vi "Save-buffered-GUI-values-to-file.vi"(8 "error in":errorcluster, 11 "Data ref. in":refnum<data-value>) -> (0 "error IO":errorcluster, 3 "Data ref.":refnum<data-value>)   [LabVIEW 2013, in "CameraVision.lvlib" / "CV-Main.lvclass"]
doc: "Saves the GUI parameter values, as currently stored in the database objects, in a number of predefined .xml files.\nAny existing files are overwritten without further warning (these checks should be performed during the file path building and communicated through the 'Proceed?' input)."
uses:
  CV-Main.lvclass
  UI/Parameters-gui.ctl
  Configuration/Configuration-parameters-gui.ctl
  Acquisition/Acquisition-parameters-gui.ctl
  Acquisition/Trigger-modes.ctl
  Acquisition/Exposure-modes.ctl
  Storage/Storage-parameters-gui.ctl
  Storage/Storage-types.ctl
  Correction/Correction-parameters-gui.ctl
  Correction/Smoothing.ctl
  Correction/Background-correction.ctl
  Analysis/Analysis-parameters-gui.ctl
  Temperature/Temperature-parameters-gui.ctl
  Mapping/Mapping-parameters-gui.ctl
  Mapping/Mapping-characteristic.ctl
  Filter/Filter-parameters-gui.ctl
  Filter/Filter-settings.ctl
  Filter/Filter-characteristic.ctl
  Filter/Filter-apply.ctl
  CV-Main.lvclass/CV-Main.ctl
  Read Acquis params.vi
  Read Analysis params.vi
  Read Config params.vi
  Read Correct params.vi
  Read Mapping params.vi
  Read Storage params.vi
  Read Temperature params.vi
  Read Filter params.vi
  Acquisition/Read-all-gui-parameters.vi
  Analysis/Read-all-gui-parameters.vi
  Configuration/Read-all-gui-params.vi
  Correction/Read-all-gui-params.vi
  Mapping/Read-all-gui-params.vi
  Storage/Read-all-gui-params.vi
  Temperature/Read-all-gui-params.vi
  Filter/Read-all-gui-parameters.vi
  <vilib>/Utility/xml.llb/Write to XML File(string).vi
  Acquisition/CV-Acquisition.lvclass
  Analysis/CV-Analysis.lvclass
  Configuration/CV-Configuration.lvclass
  Correction/CV-Correction.lvclass
  Mapping/CV-Mapping.lvclass
  Storage/CV-Storage.lvclass
  Temperature/CV-Temperature.lvclass
  Filter/CV-Filter.lvclass
  UI/CV-UI.lvclass
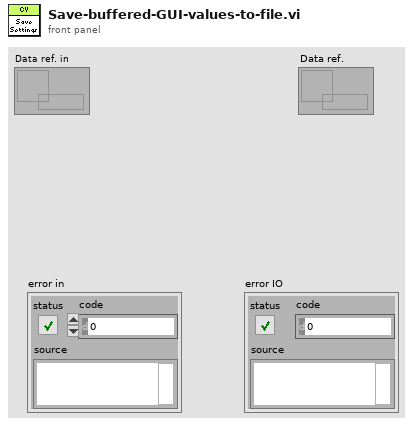
[diagram p1: front panel]
types:
  T1 = typedef "CameraVision.lvlib/CV-UI.lvclass/Parameters-gui.ctl" = cluster{"Configuration params":T2, "Acquisition params":T3, "Storage params":T6, "Correction params":T8, "Analysis params":T11, "Temperature params":T12, "Mapping params":T13, "Filter params":T15}
  T2 = typedef "CameraVision.lvlib/CV-Configuration.lvclass/Configuration-parameters-gui.ctl" = cluster{"Number of cameras":i32, "Camera 1 port":enum16{"A", "B"}, "ROI width":u32, "ROI height":u32, "Reset ROI":bool, "Width scale":dbl, "Height scale":dbl, "Center Y cam. 1":i32, "Center X cam. 1":i32, "Center Y cam. 2":i32, "Center X cam. 2":i32}
  T3 = typedef "CameraVision.lvlib/CV-Acquisition.lvclass/Acquisition-parameters-gui.ctl" = cluster{"Acquisition mode":enum16{"Continuous", "Continuous batch", "Single batch", "Single batch -delayed"}, "Batch size":i32, "Image buffer size":i32, "Trigger mode":T4, "Duration HH":sgl, "Acquisition start":enum16{"Immediate", "Post-phoned"}, "Duration SS":sgl, "Duration MM":sgl, "Start time":timestamp, "Max. frame rate":dbl, "Exposure time cam. 1":dbl, "Exposure time cam. 2":dbl, "Exposure mode":T5, "Value 1":dbl, "Value 2":dbl, "Time 1":dbl, "Time 2":dbl}
  T4 = typedef "CameraVision.lvlib/CV-Acquisition.lvclass/Trigger-modes.ctl" = enum16{"Camera timed (not sync.)", "Framegrabber timed (sync.)", "Software timed (sync.)", "External timing (sync.)", "Manual (sync.)", "Gated - camera (not sync.)", "Gated - grabber (sync.)", "Gated - software (sync.)", "Gated - external (sync.)"}
  T5 = typedef "CameraVision.lvlib/CV-Acquisition.lvclass/Exposure-modes.ctl" = enum16{"Linear", "LinLog"}
  T6 = typedef "CameraVision.lvlib/CV-Storage.lvclass/Storage-parameters-gui.ctl" = cluster{"Base file name":string, "Storage directory":path, "Save what?":T7, "Image file type":enum16{"JPG", "BMP", "PNG"}, "Comments":string, "Storage mode":enum16{"1 file per layer", "1 file for all layers "}, "Start iteration/layer":u16}
  T7 = typedef "CameraVision.lvlib/CV-Storage.lvclass/Storage-types.ctl" = cluster{"Original":bool, "Corrected":bool, "Binary":bool, "Temperature":bool, "Characteristics":bool, "Mapping":bool, "TemperatureValues":bool}
  T8 = typedef "CameraVision.lvlib/CV-Correction.lvclass/Correction-parameters-gui.ctl" = cluster{"Background correction":bool, "Hot-pixel correction":bool, "Black image cam. 1":path, "Black image cam. 2":path, "Y-shift":i32, "X-shift":i32, "Correlation algorithm":enum16{"Fixed shift", "Cross-correlation", "Cross-correlation (5steps)", "Melt-pool center"}, "Noise treshold":sgl, "Smoothing algorithm":T9, "2nd image correlation":bool, "Image smoothing":bool, "Background correction method":T10}
  T9 = typedef "CameraVision.lvlib/CV-Correction.lvclass/Smoothing.ctl" = enum16{"Noise tresholding", "NT+Median filter", "NT+Gaussian filter"}
  T10 = typedef "CameraVision.lvlib/CV-Correction.lvclass/Background-correction.ctl" = enum16{"Hardware", "Software"}
  T11 = typedef "CameraVision.lvlib/CV-Analysis.lvclass/Analysis-parameters-gui.ctl" = cluster{"Binarization treshold":sgl, "Image characteristics":bool, "Melt-pool characteristics":bool}
  T12 = typedef "CameraVision.lvlib/CV-Temperature.lvclass/Temperature-parameters-gui.ctl" = cluster{"Temperature field":bool, "Ratio correction factor":dbl, "Temperature value":bool, "Y-coord.":dbl, "X-coord.":dbl, "Averaging center":enum16{"Fixed coordinates (pixel)", "Fixed coordinates (mm)", "Melt-pool center"}, "Averaging shape":enum16{"Point", "Circle", "Ellipse"}, "Minor axis":dbl, "Major axis":dbl}
  T13 = typedef "CameraVision.lvlib/CV-Mapping.lvclass/Mapping-parameters-gui.ctl" = cluster{"Enable mapping":bool, "Automatic timing":bool, "Scan pattern file":path, "Start off-set":dbl, "Default map characteristic":T14, "Default mark speed":i32, "Jump speed":i32}
  T14 = typedef "CameraVision.lvlib/CV-Mapping.lvclass/Mapping-characteristic.ctl" = enum16{"Average intensity [0-255]", "Peak intensity [0-255]", "Melt-pool size [mm²]", "Melt-pool aspect ratio []", "Melt-pool fragments []", "Average temperature [°C]", "Max. temperature [°C]", "Min. temperature [°C]", "Std. dev. temperature [°C]"}
  T15 = typedef "CameraVision.lvlib/CV-Filter.lvclass/Filter-parameters-gui.ctl" = cluster{"Filter array":T16[], "Storage filters":T18}
  T16 = typedef "CameraVision.lvlib/CV-Filter.lvclass/Filter-settings.ctl" = cluster{"Characteristic":T17, "Monitor":bool, "Min.":dbl, "Max.":dbl, "Min. Thres.":dbl, "Min. Dur.":u16, "Report":bool}
  T17 = typedef "CameraVision.lvlib/CV-Filter.lvclass/Filter-characteristic.ctl" = enum16{"Average intensity [0-255]", "Peak intensity [0-255]", "Melt-pool size [mm²]", "Melt-pool aspect ratio []", "Melt-pool fragments []", "Melt-pool position X [pixel]", "Melt-pool position Y [pixel]", "Average temperature [°C]", "Max. temperature [°C]", "Min. temperature [°C]", "Std. dev. temperature [°C]"}
  T18 = typedef "CameraVision.lvlib/CV-Filter.lvclass/Filter-apply.ctl" = cluster{"Filter images":bool, "Filter characteristics":bool, "Filter temperature":bool}
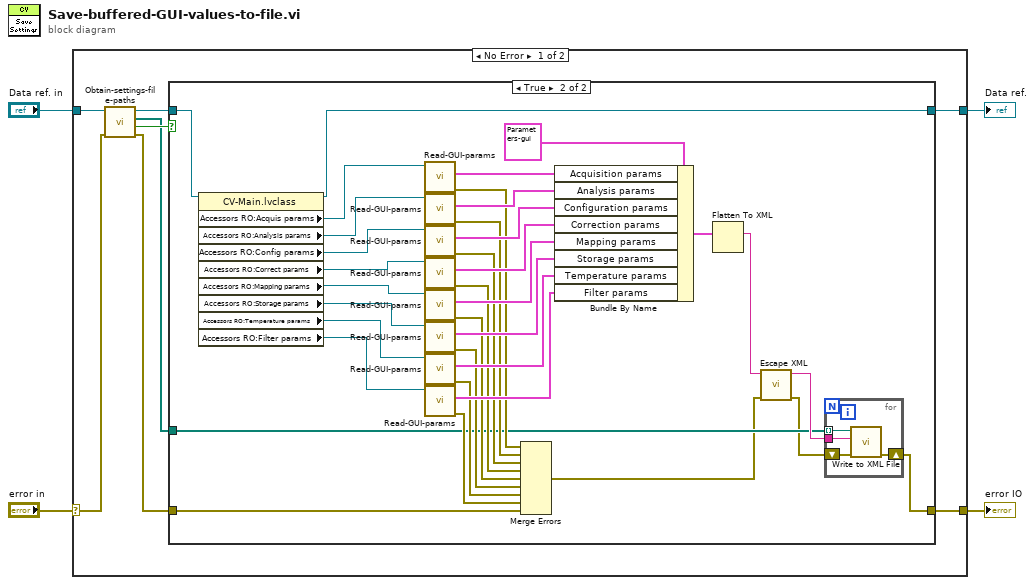
[diagram p0: block diagram]
diagram:
  n1 = case shown="No Error" "error in" {
    selector: "error in" -> [w6 w55]
    tunnel: [w12 w55] -> w4
    tunnel: "Data ref. in" -> [w10 w54]
    tunnel: [w11 w54] -> w1
    frame No Error {
      n2 = call "Obtain-settings-file-paths.vi"("error in"=w6, "Data ref. in"=w10) -> ("error IO"=w5:errorcluster, "Path ok?"=w8:bool, "File paths"=w7:path[], "Data ref."=w9:refnum<data-value>)  [unwired: 6 in]
      n3 = case shown="True" w8 {
        tunnel: w7 -> [_ w29]
        tunnel: w5 -> [w14 w15]
        tunnel: [w14 w27] -> w12
        tunnel: w9 -> [w13 w17]
        tunnel: [w13 w16] -> w11
        frame False {
        }
        frame True {
          n4 = property class="CV-Main.lvclass"(reference=w17) -> (reference out=w16:refnum<data-value>, "Accessors RO:Acquis params"=w25:refnum<data-value>, "Accessors RO:Analysis params"=w24:refnum<data-value>, "Accessors RO:Config params"=w23:refnum<data-value>, "Accessors RO:Correct params"=w22:refnum<data-value>, "Accessors RO:Mapping params"=w21:refnum<data-value>, "Accessors RO:Storage params"=w20:refnum<data-value>, "Accessors RO:Temperature params"=w19:refnum<data-value>, "Accessors RO:Filter params"=w18:refnum<data-value>)  [unwired: 1 in, 1 out]
          n5 = call-poly "Read-GUI-params.vi"("Acquis. params. ref. in"=w25) -> ("error out"=w40:errorcluster, "Acquisition params."=w48:T3)  [unwired: 8 in, 1 out]
          n6 = call-poly "Read-GUI-params.vi"("Analysis params. ref. in"=w24) -> ("error out"=w39:errorcluster, "Analys. params."=w47:T11)  [unwired: 8 in, 1 out]
          n7 = call-poly "Read-GUI-params.vi"("Config. params. ref. in"=w23) -> ("error out"=w38:errorcluster, "Configuration params."=w46:T2)  [unwired: 8 in, 1 out]
          n8 = call-poly "Read-GUI-params.vi"("Correct. params. ref. in"=w22) -> ("error out"=w37:errorcluster, "Correction params."=w45:T8)  [unwired: 8 in, 1 out]
          n9 = call-poly "Read-GUI-params.vi"("Mapping params. ref. in"=w21) -> ("error out"=w36:errorcluster, "Mapping params."=w44:T13)  [unwired: 8 in, 1 out]
          n10 = call-poly "Read-GUI-params.vi"("Storage params. ref. in"=w20) -> ("error out"=w35:errorcluster, "Storage params."=w43:T6)  [unwired: 8 in, 1 out]
          n11 = call-poly "Read-GUI-params.vi"("Temp. params. ref. in"=w19) -> ("error out"=w34:errorcluster, "Temperature params."=w42:T12)  [unwired: 8 in, 1 out]
          n12 = call-poly "Read-GUI-params.vi"("Filter params. ref. in"=w18) -> ("error IO"=w33:errorcluster, "Filter params."=w41:T15)  [unwired: 8 in, 1 out]
          n13 = Merge Errors(w40, w39, w38, w37, w36, w35, w34, w33, w15) -> (w26:errorcluster)
          n14 = Bundle By Name(cluster=T1 {"Configuration params"={"Number of cameras"=0, "Camera 1 port"=enum."B", "ROI width"=0, "ROI height"=1248, "Reset ROI"=FALSE, "Width scale"=0.0, "Height scale"=0.05, "Center Y cam. 1"=0, "Center X cam. 1"=1, "Center Y cam. 2"=1, "Center X cam. 2"=1}, "Acquisition params"={"Acquisition mode"=enum."Continuous", "Batch size"=0, "Image buffer size"=1, "Trigger mode"=enum."Camera timed (not sync.)", "Duration HH"=0.0, "Acquisition start"=enum."Post-phoned", "Duration SS"=0.01, "Duration MM"=0.01, "Start time"=timestamp(0 s since 1904-01-01), "Max. frame rate"=0.0, "Exposure time cam. 1"=0.0, "Exposure time cam. 2"=0.0, "Exposure mode"=enum."Linear", "Value 1"=0.0, "Value 2"=0.0, "Time 1"=0.0, "Time 2"=0.0}, "Storage params"={"Base file name"="", "Storage directory"=path "", "Save what?"={"Original"=FALSE, "Corrected"=FALSE, "Binary"=FALSE, "Temperature"=FALSE, "Characteristics"=FALSE, "Mapping"=FALSE, "TemperatureValues"=FALSE}, "Image file type"=enum."BMP", "Comments"="", "Storage mode"=enum."1 file per layer", "Start iteration/layer"=0}, "Correction params"={"Background correction"=FALSE, "Hot-pixel correction"=FALSE, "Black image cam. 1"=path "", "Black image cam. 2"=path "", "Y-shift"=0, "X-shift"=0, "Correlation algorithm"=enum."Fixed shift", "Noise treshold"=0.0, "Smoothing algorithm"=enum."Noise tresholding", "2nd image correlation"=FALSE, "Image smoothing"=FALSE, "Background correction method"=enum."Hardware"}, "Analysis params"={"Binarization treshold"=0.0, "Image characteristics"=FALSE, "Melt-pool characteristics"=FALSE}, "Temperature params"={"Temperature field"=FALSE, "Ratio correction factor"=0.0, "Temperature value"=FALSE, "Y-coord."=0.0, "X-coord."=0.0, "Averaging center"=enum."Fixed coordinates (pixel)", "Averaging shape"=enum."Point", "Minor axis"=0.0, "Major axis"=0.0}, "Mapping params"={"Enable mapping"=FALSE, "Automatic timing"=FALSE, "Scan pattern file"=path "", "Start off-set"=40.0, "Default map characteristic"=enum."Average intensity [0-255]", "Default mark speed"=0, "Jump speed"=0}, "Filter params"={"Filter array"=[], "Storage filters"={"Filter images"=FALSE, "Filter characteristics"=FALSE, "Filter temperature"=FALSE}}} ("Parameters"), "Acquisition params"=w48, "Analysis params"=w47, "Configuration params"=w46, "Correction params"=w45, "Mapping params"=w44, "Storage params"=w43, "Temperature params"=w42, "Filter params"=w41) -> (w31:T1)
          n15 = Flatten To XML(anything=w31) -> (xml string=w32:string)
          n16 = call <vilib>:"Escape XML.vi"("error in (no error)"=w26, "XML String In"=w32) -> ("error out"=w28:errorcluster, "XML String Out"=w30:string)  [unwired: 8 in]
          n17 = for {
            tunnel: w30 -> [w53]
            tunnel: w29 -> [w52] mode=indexing
            shift-right: [w50] -> w27
            shift-left: w28 -> [w51]
            n18 = call-poly <vilib>:"Write to XML File.vi"("error in (no error)"=w51, "XML Input"=w53, "XML File Path"=w52) -> ("error out"=w50:errorcluster)  [unwired: 6 in, 2 out]
          }
        }
      }
    }
    frame Error {
    }
  }
  "error IO" <- w4
  "Data ref." <- w1
